vi "Write Strings And Values [].vi"(8 "error in (no error)":errorcluster, 10 "StringsAndValues[]":T1, 11 "Ring.lvclass in":refnum<class "Ring.lvclass">) -> (0 "error out":errorcluster, 3 "Ring.lvclass out":refnum<class "Ring.lvclass">)   [LabVIEW 2015, in "Ring.lvclass"]
uses:
  Ring.lvclass
  <vilib>/Utility/miscctls.llb/LVStringsAndValuesArrayTypeDef.ctl
  Ring.lvclass/Ring.ctl
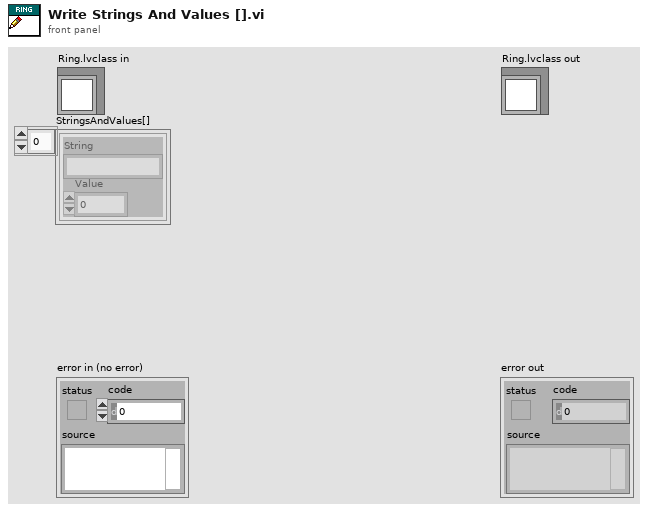
[diagram p1: front panel]
types:
  T1 = typedef "LVStringsAndValuesArrayTypeDef.ctl" = cluster{"String":string, "Value":ext}[]
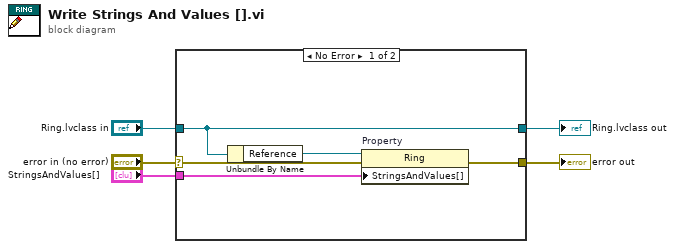
[diagram p0: block diagram]
diagram:
  n1 = case shown="No Error" "error in (no error)" {
    selector: "error in (no error)" -> [w6 w12]
    tunnel: [w10 w12] -> w4
    tunnel: [w8 w11] -> w2
    tunnel: "Ring.lvclass in" -> [w8 w11]
    tunnel: "StringsAndValues[]" -> [w9 _]
    frame No Error {
      n2 = Unbundle By Name(w8) -> ("Reference"=w7:refnum<vi>)
      n3 = property on="Property" class="Ring"(reference=w7, error in=w6, "StringsAndValues[]"=w9) -> (error out=w10:errorcluster)  [unwired: 1 out]
    }
    frame Error {
    }
  }
  "error out" <- w4
  "Ring.lvclass out" <- w2
